vi "Target CSM.vi"(5 "Init State(\"Macro: Initialize\")":string="Macro: Initialize", 7 "Name(\"\" to use uuid)":string="CSM Tiny") -> ()   [LabVIEW 2020]
doc: "Template for building CSM Module without User Interface.\n\n<b>Inputs:</b>\n- <b>Name(\"\" to use uuid)</b>: Module Name\n - If Input is \"\", an uuid will be used for module name. The module is marked as stand-alone mode and will not be included in module list.\n - Fi Input end with '#', the module will worked in worker mode. Modules with the same name will shared the same message queue. Any external message will be processed by one of the modules, depends on who is free.\n - Otherwise, the input string will be used as module name, which should be unique in system. CSM will go to \"Critical Error\" state if duplicated module name is used in system.\n\n<b>Outputs:</b>\n - N/A"
uses:
  <userlib>/_NEVSTOP/Communicable State Machine(CSM)/_Support/Priority Queue/Priority Queue.lvclass/Priority Queue.ctl
  <userlib>/_NEVSTOP/Communicable State Machine(CSM)/AdvanceAPI/CSM - Revert Arguments-Safe String.vi
  <userlib>/_NEVSTOP/Communicable State Machine(CSM)/_Support/Common/Trim Single line Text.vi
  <userlib>/_NEVSTOP/Communicable State Machine(CSM)/AdvanceAPI/CSM - Break Down Multiple States String.vi
  <userlib>/_NEVSTOP/Communicable State Machine(CSM)/AdvanceAPI/CSM - Compact Multiple States.vi
  <userlib>/_NEVSTOP/Communicable State Machine(CSM)/AdvanceAPI/CSM - Make String Arguments Safe.vi
  <userlib>/_NEVSTOP/Communicable State Machine(CSM)/_Support/Process/CSMP-Async Call.vi
  <userlib>/_NEVSTOP/Communicable State Machine(CSM)/_Support/GlobalEvent/GEvt-Generate Status Log.vi
  <userlib>/_NEVSTOP/Communicable State Machine(CSM)/_Support/Process/CSMP-Broadcast.vi
  <userlib>/_NEVSTOP/Communicable State Machine(CSM)/_Support/GlobalEvent/GEvt-Generate Interrupt Log.vi
  <userlib>/_NEVSTOP/Communicable State Machine(CSM)/_Support/GlobalEvent/GEvt-Generate Register Log.vi
  <userlib>/_NEVSTOP/Communicable State Machine(CSM)/_Support/Process/CSMP-Register Status.vi
  <userlib>/_NEVSTOP/Communicable State Machine(CSM)/_Support/GlobalEvent/GEvt-Generate Unregister Log.vi
  <userlib>/_NEVSTOP/Communicable State Machine(CSM)/_Support/Process/CSMP-Unregister Status.vi
  <userlib>/_NEVSTOP/Communicable State Machine(CSM)/_Support/Process/CSMP-Sync Call.vi
  <userlib>/_NEVSTOP/Communicable State Machine(CSM)/_Support/CSMQ/_CSMObj-Unlock.vi
  <userlib>/_NEVSTOP/Communicable State Machine(CSM)/_Support/Process/CSMP-PostPostMsg.vi
  <userlib>/_NEVSTOP/Communicable State Machine(CSM)/_Support/Process/CSMP-PostSendMsg.vi
  <userlib>/_NEVSTOP/Communicable State Machine(CSM)/_Support/CSMQ/_CSMObj-Lock State.vi
  <userlib>/_NEVSTOP/Communicable State Machine(CSM)/_Support/Common/Splite Reason String Part.vi
  <userlib>/_NEVSTOP/Communicable State Machine(CSM)/_Support/CSMQ/_CSMOFGV Release.vi
  <userlib>/_NEVSTOP/Communicable State Machine(CSM)/_Support/Common/Remove Comments from Line.vi
  <userlib>/_NEVSTOP/Communicable State Machine(CSM)/_Support/Common/Splite Single-line Message.vi
  <userlib>/_NEVSTOP/Communicable State Machine(CSM)/_Support/Common/Parse Next Single-line State.vi
  <userlib>/_NEVSTOP/Communicable State Machine(CSM)/_Support/CSMQ/_CSMOFGV Dequeue.vi
  <userlib>/_NEVSTOP/Communicable State Machine(CSM)/_Support/CSMQ/_CSMObj-Log Error if in a Remote Session.vi
  <userlib>/_NEVSTOP/Communicable State Machine(CSM)/_Support/GlobalEvent/GEvt-Generate State Change Log.vi
  <userlib>/_NEVSTOP/Communicable State Machine(CSM)/_Support/GlobalEvent/GEvt-Generate Remaining States Log.vi
  <userlib>/_NEVSTOP/Communicable State Machine(CSM)/_Support/GlobalEvent/GEvt-Generate Module Destroyed Log.vi
  <userlib>/_NEVSTOP/Communicable State Machine(CSM)/_Support/GlobalEvent/GEvt-Generate Complete Log.vi
  <userlib>/_NEVSTOP/Communicable State Machine(CSM)/_Support/GlobalEvent/GEvt-Generate Module Created Log.vi
  <userlib>/_NEVSTOP/Communicable State Machine(CSM)/_Support/GlobalEvent/Cache-GEvt Filter Object.vi
  <userlib>/_NEVSTOP/Communicable State Machine(CSM)/_Support/Common/Format Timestamp.vi
  <userlib>/_NEVSTOP/Communicable State Machine(CSM)/AdvanceAPI/CSM - Keywords.vi
  <userlib>/_NEVSTOP/Communicable State Machine(CSM)/_Support/CSMQ/_CSMObj-Message Check.vi
  <userlib>/_NEVSTOP/Communicable State Machine(CSM)/_Support/CSMQ/_CSMObj-Enqueue Cross-Module Message.vi
  <userlib>/_NEVSTOP/Communicable State Machine(CSM)/_Support/CSMQ/_CSMOFGV Get.vi
  <userlib>/_NEVSTOP/Communicable State Machine(CSM)/_Support/GlobalEvent/GEvt-Generate with Rule Check.vi
  <userlib>/_NEVSTOP/Communicable State Machine(CSM)/_Support/FGV-BroadcastRegistry/Cache-Broadcast Registry Search Result.vi
  <userlib>/_NEVSTOP/Communicable State Machine(CSM)/AdvanceAPI/CSM - Register Status Change.vi
  <userlib>/_NEVSTOP/Communicable State Machine(CSM)/AdvanceAPI/CSM - Unregister Status Change.vi
  <userlib>/_NEVSTOP/Communicable State Machine(CSM)/_Support/Common/Hex Str to U8 Data.vi
  <userlib>/_NEVSTOP/Communicable State Machine(CSM)/_Support/Common/Concatenate State with Arguments.vi
  <userlib>/_NEVSTOP/Communicable State Machine(CSM)/_Support/Common/U8 Data to Hex Str.vi
  <userlib>/_NEVSTOP/Communicable State Machine(CSM)/_Support/Priority Queue/Dequeue Element.vi
  <userlib>/_NEVSTOP/Communicable State Machine(CSM)/_Support/Priority Queue/Enqueue Element.vi
  <userlib>/_NEVSTOP/Communicable State Machine(CSM)/_Support/GlobalEvent/LogFilter/Filter Check.vi
  <userlib>/_NEVSTOP/Communicable State Machine(CSM)/Utility/Trim Both Whitespace.vi
  <userlib>/_NEVSTOP/Communicable State Machine(CSM)/_Support/GlobalEvent/FGV-GlobalEventRef.vi
  <userlib>/_NEVSTOP/Communicable State Machine(CSM)/_Support/GlobalEvent/global-GEvnt Filter Change Flag.vi
  <userlib>/_NEVSTOP/Communicable State Machine(CSM)/FGV-GEvt Filter Obj.vi
  <userlib>/_NEVSTOP/Communicable State Machine(CSM)/_Support/CSMQ/_CSMOFGV Obtain.vi
  <userlib>/_NEVSTOP/Communicable State Machine(CSM)/_Support/GlobalEvent/LogFilter/CheckVIs/Group Check - CSM.vi
  <userlib>/_NEVSTOP/Communicable State Machine(CSM)/_Support/GlobalEvent/LogFilter/CheckVIs/Group Check - LogType.vi
  <userlib>/_NEVSTOP/Communicable State Machine(CSM)/_Support/GlobalEvent/LogFilter/CheckVIs/Group Check - State.vi
  <userlib>/_NEVSTOP/Communicable State Machine(CSM)/_Support/GlobalEvent/LogFilter/CheckVIs/CSM Check - LogType.vi
  <userlib>/_NEVSTOP/Communicable State Machine(CSM)/_Support/GlobalEvent/LogFilter/CheckVIs/CSM Check - State.vi
  <userlib>/_NEVSTOP/Communicable State Machine(CSM)/_Support/GlobalEvent/LogFilter/CheckVIs/CSM Check - StateType.vi
  <userlib>/_NEVSTOP/Communicable State Machine(CSM)/_Support/GlobalEvent/LogFilter/CheckVIs/Group Check - StateType.vi
  <userlib>/_NEVSTOP/Communicable State Machine(CSM)/_Support/CSMQ/_CSMOFGV.vi
  <userlib>/_NEVSTOP/Communicable State Machine(CSM)/_Support/Error/CSM Not Allowed Message.vi
  <userlib>/_NEVSTOP/Communicable State Machine(CSM)/_Support/GlobalEvent/FGV-StatusChangeEventRef.vi
  <userlib>/_NEVSTOP/Communicable State Machine(CSM)/_Support/FGV-BroadcastRegistry/global-CSMQ FGV Change Flag.vi
  <userlib>/_NEVSTOP/Communicable State Machine(CSM)/_Support/FGV-BroadcastRegistry/global-Broadcast Cache Change Flag.vi
  <userlib>/_NEVSTOP/Communicable State Machine(CSM)/_Support/BroadcastRegistry/HelperVI/Broadcast Item Key.vi
  <userlib>/_NEVSTOP/Communicable State Machine(CSM)/_Support/FGV-BroadcastRegistry/FGV-BroadcastRegistry.vi
  <userlib>/_NEVSTOP/Communicable State Machine(CSM)/_Support/Message/Parse Register Message.vi
  <userlib>/_NEVSTOP/Communicable State Machine(CSM)/_Support/Message/Parse Unregister Message.vi
  <userlib>/_NEVSTOP/Communicable State Machine(CSM)/Communicable State Machine.lvlib
panel:
  out "State History":string
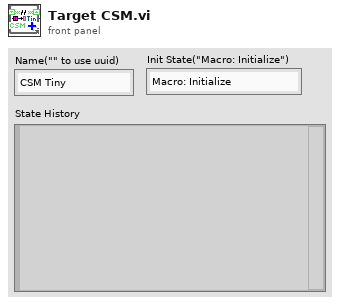
[diagram p1: front panel]
types:
  T1 = enum32{"Invalid", "Standard", "Closed", "Hidden", "Minimized", "Maximized"}
  T2 = enum32{"invalid app kind", "Development System", "Run Time System", "Student Edition", "Embedded LabVIEW", "Evaluation", "Custom"}
  T3 = typedef "Communicable State Machine.lvlib/_CSM_Response Source Message.ctl" = cluster{"‘State":string, "’Arguments":string, "’Error":errorcluster}
  T4 = cluster{"Current VI Reference":refnum<vi>, "Close Panel on Exit?":bool}
  T5 = cluster{"Core":cluster{"Current VI Reference":refnum<vi>, "Close Panel on Exit?":bool}, "Your Boolean data":bool, "Your string data":string}
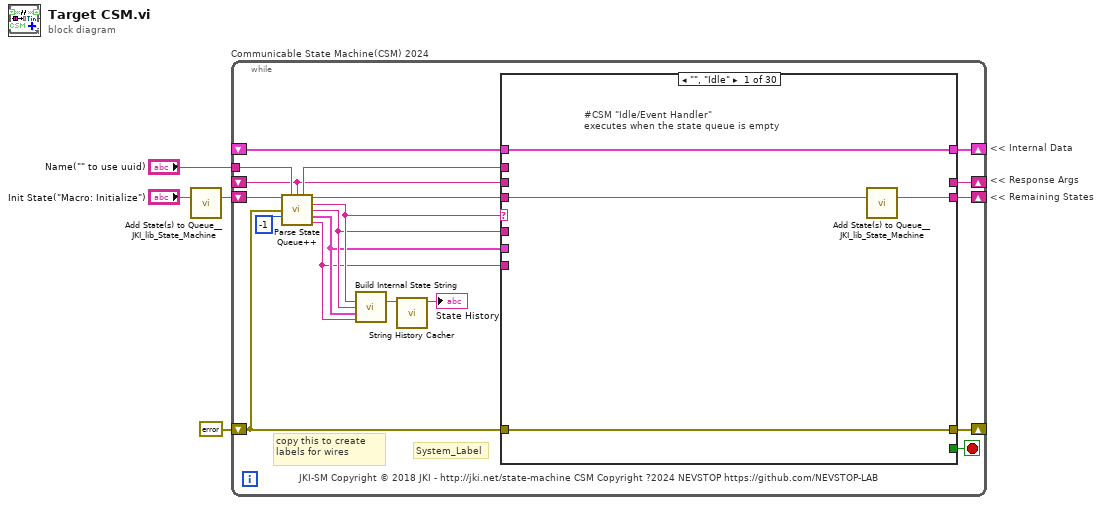
[diagram p0: block diagram]
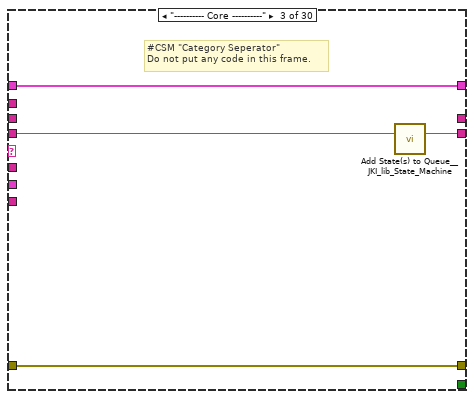
[diagram p3: hidden frame]
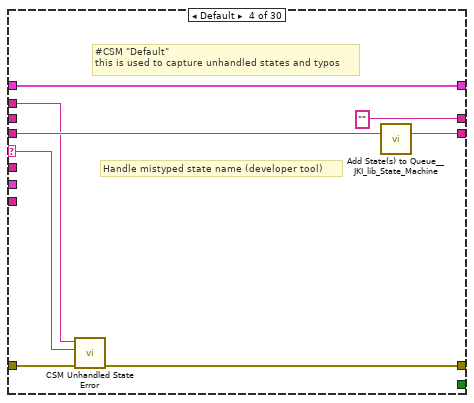
[diagram p4: hidden frame]
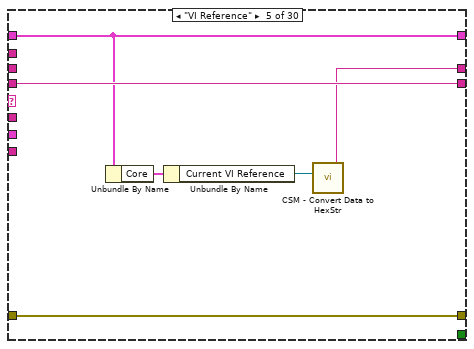
[diagram p5: hidden frame]
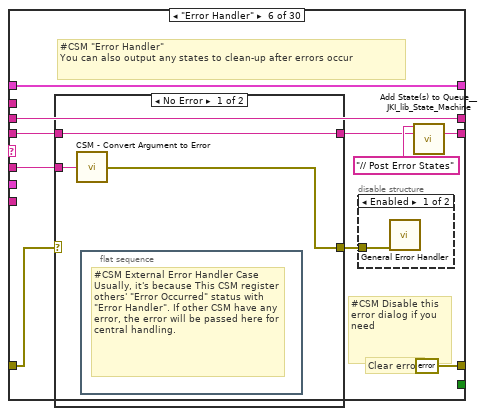
[diagram p6: hidden frame]
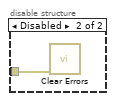
[diagram p7: hidden frame]
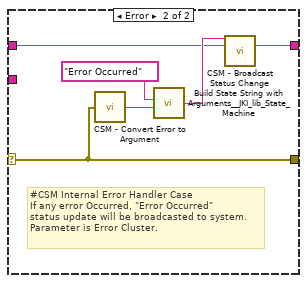
[diagram p8: hidden frame]
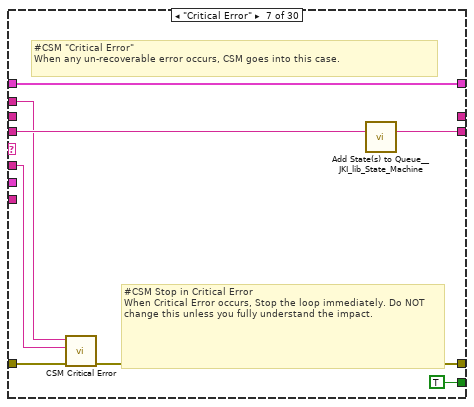
[diagram p9: hidden frame]
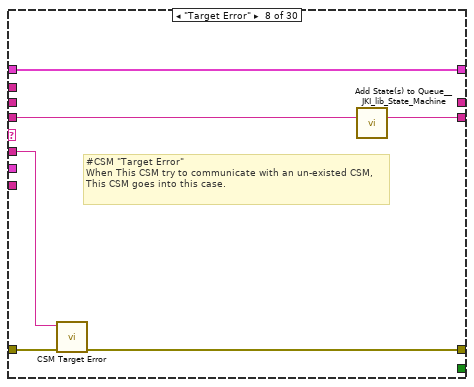
[diagram p10: hidden frame]
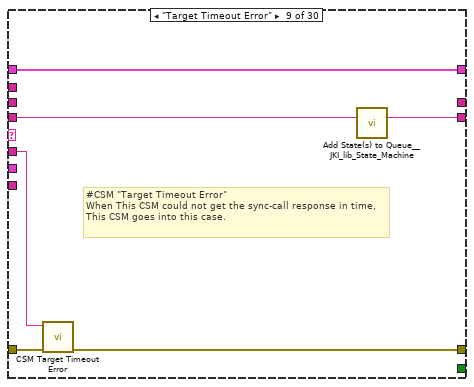
[diagram p11: hidden frame]
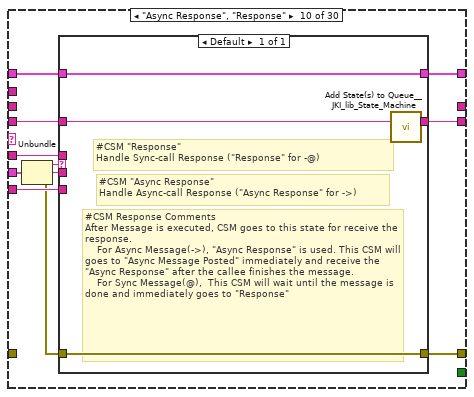
[diagram p12: hidden frame]
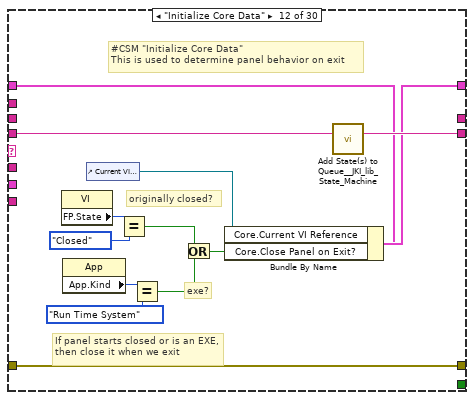
[diagram p14: hidden frame]
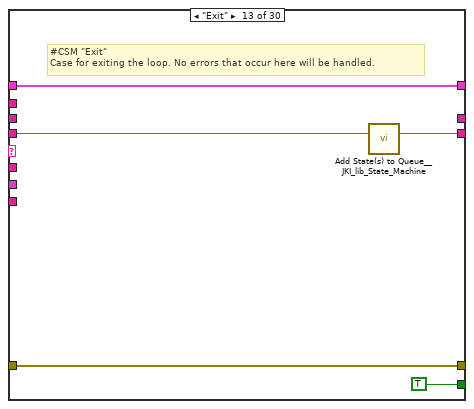
[diagram p15: hidden frame]
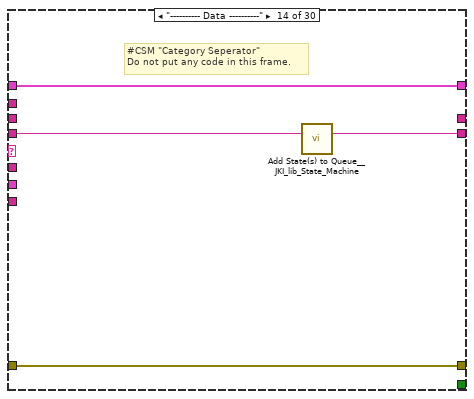
[diagram p16: hidden frame]
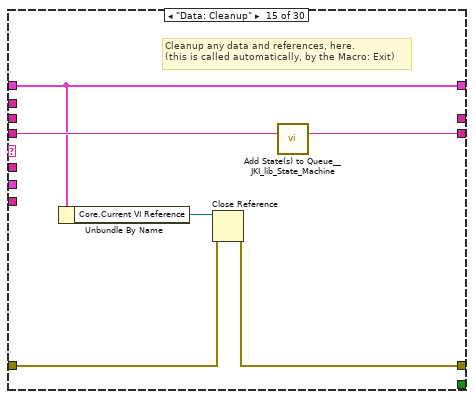
[diagram p17: hidden frame]
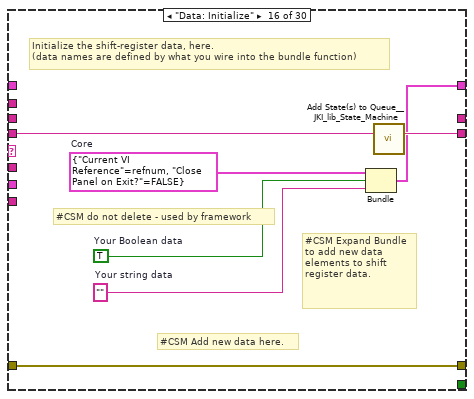
[diagram p18: hidden frame]
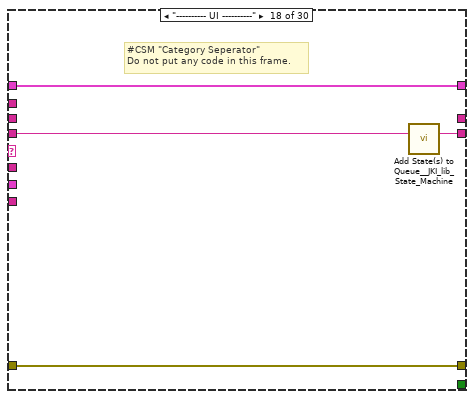
[diagram p20: hidden frame]
diagram:
  # "<< Internal Data"
  # "<< Response Args"
  # "<< Remaining States"
  n1 = call <vilib>:"Add State(s) to Queue__JKI_lib_State_Machine.vi"("State(s) in (\"\")"="Init State(\"Macro: Initialize\")") -> ("States Out"=w4:string)  [unwired: 14 in]
  n2 = while "Communicable State Machine(CSM) 2024" {
    shift-right: [w18] -> _
    shift-left: _ -> [w17]
    shift-right: [w21] -> _
    shift-left: errorcluster {"status"=FALSE, "code"=0, "source"=""} ("error out") -> [w16]
    shift-right: [w20] -> _
    shift-left: w4 -> [w22]
    tunnel: "Name(\"\" to use uuid)" -> [w14]
    shift-right: [w15] -> _
    shift-left: _ -> [w6]
    stop <- w19 stop-if-true
    # "copy this to create labels for wires"
    # "System_Label"
    # "JKI-SM Copyright © 2018 JKI - http://jki.net/state-machine CSM Copyright ?2024 NEVSTOP https://github.com/NEVSTOP-LAB"
    n3 = call <userlib>:"Parse State Queue++.vi"("State Queue"=w22, "Name(\"\" to use uuid)"=w14, "Response Arguments"=w6, "Error In (no error)"=w16, "Dequeue Timeout(0ms)"=-1 ("Timeout")) -> ("Name Used"=w7:string, "Remaining States"=w23:string, "Current State"=w11:string, "Arguments"=w10:string, ">> Response Source Message >>"=w9:T3, ">> Source CSM >>"=w8:string)  [unwired: 5 in]
    n4 = call <userlib>:"Build Internal State String.vi"("State"=w11, "Arguments (\"\")"=w10, ">> Response Source Message >>"=w9, "Source (\"\")"=w8) -> ("State with Arguments"=w12:string)  [unwired: 11 in]
    n5 = call <userlib>:"String History Cacher.vi"("String"=w12) -> ("String Cache"=→"State History":string)  [unwired: 10 in]
    n6 = case shown="\"\", \"Idle\"" w11 {
      selector: w11 -> [_ _ _ w37 _ _ _ _ _ _ _ _ _ _ _ _ _ _ _ _ _ _ _ _ _ _ _ _ _ _]
      tunnel: w23 -> [w24 w29 w34 w41 w47 w54 w75 w81 w87 w95 w106 w120 w125 w129 w135 w142 w144 w149 w153 w159 w174 w243 w248 w255 w257 w262 w268 w273 w277 w281]
      tunnel: w10 -> [_ _ _ _ _ w53 w71 w80 w85 w94 _ _ _ _ _ _ _ _ _ w154 w168 _ _ _ _ w260 _ _ _ _]
      tunnel: w17 -> [w25 w28 w31 w39 w46 w57 w76 w82 w88 w97 w105 w113 w123 w126 w130 _ w143 w146 w151 w157 w170 w240 w245 w252 w256 w261 w267 w270 w274 w278]
      tunnel: [w26 w30 w32 w35 w48 errorcluster {"status"=FALSE, "code"=0, "source"=""} ("error out") w72 w78 w84 w100 w107 w117 w122 w127 w131 w139 w145 w147 w150 w155 w171 w241 w246 w253 w258 w263 w269 w271 w275 w279] -> w21
      tunnel: w16 -> [w26 w30 w32 w42 w48 w55 w77 w79 w86 _ w107 w117 w122 w127 w132 w139 w145 w147 w150 w156 w172 w241 w246 w253 w258 w263 w269 w271 w275 w279]
      tunnel: [w27 w29 w33 w40 w47 w50 w74 w83 w89 w96 w106 w119 w124 w128 w134 w141 w144 w148 w152 w158 w173 w242 w247 w254 w257 w262 w268 w272 w276 w280] -> w20
      tunnel: [_ _ _ _ _ _ TRUE _ _ _ _ _ TRUE _ _ _ _ _ _ _ _ _ _ _ _ _ _ _ _ _] -> w19
      tunnel: [w25 w28 w31 w39 w46 w57 w76 w82 w88 w98 w105 w118 w123 w126 w130 w140 w143 w146 w151 w157 w170 w240 w245 w252 w256 w261 w267 w270 w274 w278] -> w18
      tunnel: w8 -> [_ _ _ _ _ _ _ _ _ w92 _ _ _ _ _ _ _ _ _ _ _ _ _ _ _ _ _ _ _ _]
      tunnel: w9 -> [_ _ _ _ _ _ _ _ _ w99 _ _ _ _ _ _ _ _ _ _ _ _ _ _ _ _ _ _ _ _]
      tunnel: [_ _ _ "" w43 w49 _ _ _ _ _ _ _ _ _ _ _ _ _ _ _ _ _ _ _ w259 "API1 Response" _ _ _] -> w15
      tunnel: w7 -> [_ _ _ w36 _ _ w70 _ _ _ _ _ _ _ _ _ _ _ _ _ _ _ _ _ _ _ _ _ _ _]
      tunnel: w6 -> [_ _ _ _ _ w49 _ _ _ _ _ _ _ _ _ _ _ _ _ _ _ _ _ _ _ _ _ _ _ _]
      frame "", "Idle" {
        # "#CSM \"Idle/Event Handler\"\nexecutes when the state queue is empty"
        n7 = call <vilib>:"Add State(s) to Queue__JKI_lib_State_Machine.vi"("State(s) in (\"\")"=w24) -> ("States Out"=w27:string)  [unwired: 14 in]
      }
      frame "CSM Documentation" {
        # "#CSM README FIRST\n\nCommunicable State Machine(CSM) is a LabVIEW application framework that builds upon JKI State Machine(JKISM). It follows the pattern of JKISM and extends the keywords to describe message communication between modules, including concepts such as Sync-Message, Async-Message, Subscription/Unsubscription of status - essential elements for creating reusable code modules. For more information, please visit the CSM wiki: https://nevstop-lab.github.io/CSM-Wiki/\n\nFor instructions on JKI State Machine, visit: http://jki.net/state-machine/\nFor information about CSM, visit: https://github.com/NEVSTOP-LAB"
        # "#CSM \"Documentation\"\nCase for holding CSM Documenation"
      }
      frame "---------- Core ----------" {
        # "#CSM \"Category Seperator\"\nDo not put any code in this frame."
        n8 = call <vilib>:"Add State(s) to Queue__JKI_lib_State_Machine.vi"("State(s) in (\"\")"=w34) -> ("States Out"=w33:string)  [unwired: 14 in]
      }
      frame Default {
        # "#CSM \"Default\"\nthis is used to capture unhandled states and typos"
        # "Handle mistyped state name (developer tool)"
        n9 = call <userlib>:"CSM Unhandled State Error.vi"("error in (no error)"=w42, "Current State"=w37, "CSM Name"=w36) -> ("error out"=w35:errorcluster)  [unwired: 8 in]
        n10 = call <vilib>:"Add State(s) to Queue__JKI_lib_State_Machine.vi"("State(s) in (\"\")"=w41) -> ("States Out"=w40:string)  [unwired: 14 in]
      }
      frame "VI Reference" {
        n11 = Unbundle By Name(w46) -> ("Core"=w45:T4)
        n12 = Unbundle By Name(w45) -> ("Current VI Reference"=w44:refnum<vi>)
        n13 = call <userlib>:"CSM - Convert Data to HexStr.vi"("Variant"=w44) -> ("HEX String (0-9,A-F)"=w43:string)  [unwired: 8 in]
      }
      frame "Error Handler" {
        # "#CSM Disable this error dialog if you need"
        # "#CSM \"Error Handler\"\nYou can also output any states to clean-up after errors occur"
        # "Clear error"
        n14 = case shown="No Error" w55 {
          selector: w55 -> [_ w64]
          tunnel: [w63 w66] -> w51
          tunnel: w54 -> [w63 w65]
          tunnel: w53 -> [w62 _]
          tunnel: [w61 w64] -> w56
          frame No Error {
            n15 = call <userlib>:"CSM - Convert Argument to Error.vi"("Argument"=w62) -> ("error"=w61:errorcluster)  [unwired: 4 in]
            n16 = flat-sequence {
              frame #0 {
                # "#CSM External Error Handler Case\nUsually, it's because This CSM register others' \"Error Occurred\" status with \"Error Handler\". If other CSM have any error, the error will be passed here for central handling."
              }
            }
          }
          frame Error {
            # "#CSM Internal Error Handler Case \nIf any error Occurred, \"Error Occurred\" \nstatus update will be broadcasted to system.\nParameter is Error Cluster."
            n17 = call <userlib>:"CSM - Convert Error to Argument.vi"("error in (no error)"=w64) -> ("Arguments"=w68:string)  [unwired: 4 in]
            n18 = call <vilib>:"Build State String with Arguments__JKI_lib_State_Machine.vi"("Arguments (\"\")"=w68, "State"="Error Occurred" ("Status with Arguments")) -> ("State with Arguments"=w67:string)  [unwired: 4 in]
            n19 = call <userlib>:"CSM - Broadcast Status Change.vi"("Status with Arguments"=w67, "State Queue"=w65) -> ("Remaining States"=w66:string)  [unwired: 13 in]
          }
        }
        n20 = disable-structure shown="Enabled" {
          disable-tunnel: w56 -> [w59 w60]
          frame Enabled {
            n21 = call <vilib>:"General Error Handler.vi"("error in (no error)"=w59) -> ()  [unwired: 10 in, 5 out]
          }
          frame Disabled {
            n22 = call <vilib>:"Clear Errors.vi"("error in (no error)"=w60) -> ()  [unwired: 5 in, 2 out]
          }
        }
        n23 = call <vilib>:"Add State(s) to Queue__JKI_lib_State_Machine.vi"("State(s) in Front (\"\")"="// Post Error States", "State(s) in (\"\")"=w51) -> ("States Out"=w50:string)  [unwired: 13 in]
      }
      frame "Critical Error" {
        # "#CSM Stop in Critical Error\nWhen Critical Error occurs, Stop the loop immediately. Do NOT change this unless you fully understand the impact."
        # "#CSM \"Critical Error\"\nWhen any un-recoverable error occurs, CSM goes into this case."
        n24 = call <userlib>:"CSM Critical Error.vi"("error in (no error)"=w77, "Arugments(as Reason)"=w71, "CSM Name"=w70) -> ("error out"=w72:errorcluster)  [unwired: 8 in]
        n25 = call <vilib>:"Add State(s) to Queue__JKI_lib_State_Machine.vi"("State(s) in (\"\")"=w75) -> ("States Out"=w74:string)  [unwired: 14 in]
      }
      frame "Target Error" {
        # "#CSM \"Target Error\"\nWhen This CSM try to communicate with an un-existed CSM, This CSM goes into this case."
        n26 = call <userlib>:"CSM Target Error.vi"("error in (no error)"=w79, "Arguments(as CSM Name)"=w80) -> ("error out"=w78:errorcluster)  [unwired: 9 in]
        n27 = call <vilib>:"Add State(s) to Queue__JKI_lib_State_Machine.vi"("State(s) in (\"\")"=w81) -> ("States Out"=w83:string)  [unwired: 14 in]
      }
      frame "Target Timeout Error" {
        # "#CSM \"Target Timeout Error\"\nWhen This CSM could not get the sync-call response in time, This CSM goes into this case."
        n28 = call <userlib>:"CSM Target Timeout Error.vi"("error in (no error)"=w86, "Arguments(as CSM Name)"=w85) -> ("error out"=w84:errorcluster)  [unwired: 9 in]
        n29 = call <vilib>:"Add State(s) to Queue__JKI_lib_State_Machine.vi"("State(s) in (\"\")"=w87) -> ("States Out"=w89:string)  [unwired: 14 in]
      }
      frame "Async Response", "Response" {
        n30 = Unbundle(w99) -> ("‘State"=w93:string, "’Arguments"=w91:string, "’Error"=w90:errorcluster)
        n31 = case shown="Default" w93 {
          tunnel: [w104] -> w100
          tunnel: w90 -> [w104]
          tunnel: [w103] -> w98
          tunnel: w97 -> [w103]
          tunnel: [w101] -> w96
          tunnel: w95 -> [w102]
          tunnel: w94 -> [_]
          tunnel: w92 -> [_]
          tunnel: w91 -> [_]
          frame Default {
            # "#CSM Response Comments\nAfter Message is executed, CSM goes to this state for receive the response.\n    For Async Message(->), \"Async Response\" is used. This CSM will goes to \"Async Message Posted\" immediately and receive the \"Async Response\" after the callee finishes the message.\n    For Sync Message(@),  This CSM will wait until the message is done and immediately goes to \"Response\""
            # "#CSM \"Async Response\"\nHandle Async-call Response (\"Async Response\" for ->)"
            # "#CSM \"Response\"\nHandle Sync-call Response (\"Response\" for -@)"
            n32 = call <vilib>:"Add State(s) to Queue__JKI_lib_State_Machine.vi"("State(s) in (\"\")"=w102) -> ("States Out"=w101:string)  [unwired: 14 in]
          }
        }
      }
      frame "Async Message Posted" {
        # "a"
        # "a"
        # "a"
        # "a"
        # "a"
        # "a"
        # "a"
        # "a"
        # "a"
        # "a"
        # "a"
        # "a"
        # "a"
        # "a"
        # "a"
        # "a"
        # "a"
        # "a"
        # "a"
        # "a"
        # "a"
        # "a"
        # "a"
        # "a"
        # "a"
        # "a"
        # "a"
        # "a"
        # "a"
        # "a"
        # "a"
        # "a"
        # "a"
        # "a"
        # "a"
        # "a"
        # "a"
        # "a"
        # "a"
        # "a"
        # "a"
        # "a"
        # "a"
        # "a"
        # "a"
        # "a"
        # "a"
        # "a"
        # "a"
        # "a"
        # "a"
        # "a"
        # "a"
        # "a"
        # "a"
        # "a"
        # "a"
        # "a"
        # "a"
        # "a"
        # "a"
        # "a"
        # "a"
        # "a"
        # "a"
        # "a"
        # "a"
        # "a"
        # "a"
        # "a"
        # "a"
        # "a"
        # "a"
        # "a"
        # "a"
        # "a"
        # "a"
        # "a"
        # "a"
        # "a"
        # "a"
        # "a"
        # "a"
        # "a"
        # "a"
        # "a"
        # "a"
        # "a"
        # "a"
        # "a"
        # "a"
        # "a"
        # "a"
        # "a"
        # "a"
        # "a"
        # "a"
        # "a"
        # "a"
        # "a"
        # "a"
        # "a"
        # "a"
        # "a"
        # "a"
        # "a"
        # "a"
        # "a"
        # "a"
        # "a"
        # "a"
        # "a"
        # "a"
        # "a"
        # "a"
        # "a"
        # "a"
        # "a"
        # "a"
        # "a"
        # "a"
        # "a"
        # "a"
        # "a"
        # "a"
        # "a"
        # "a"
        # "a"
        # "a"
        # "a"
        # "a"
        # "a"
        # "a"
        # "a"
        # "a"
        # "a"
        # "a"
        # "a"
        # "a"
        # "a"
        # "a"
        # "a"
        # "a"
        # "a"
        # "a"
        # "a"
        # "a"
        # "a"
        # "a"
        # "a"
        # "a"
        # "a"
        # "a"
        # "a"
        # "a"
        # "a"
        # "a"
        # "a"
        # "a"
        # "a"
        # "a"
        # "a"
        # "a"
        # "a"
        # "a"
        # "a"
        # "a"
        # "a"
        # "a"
        # "a"
        # "a"
        # "a"
        # "a"
        # "a"
        # "a"
        # "a"
        # "a"
        # "a"
        # "a"
        # "a"
        # "a"
        # "a"
        # "a"
        # "a"
        # "a"
        # "a"
        # "a"
        # "a"
        # "a"
        # "a"
        # "a"
        # "a"
        # "a"
        # "a"
        # "a"
        # "a"
        # "a"
        # "a"
        # "a"
        # "a"
        # "a"
        # "a"
        # "a"
        # "a"
        # "a"
        # "a"
        # "a"
        # "a"
        # "a"
        # "a"
        # "a"
        # "a"
        # "a"
        # "a"
        # "a"
        # "a"
        # "a"
        # "a"
        # "a"
        # "a"
        # "a"
        # "a"
        # "a"
        # "a"
        # "a"
        # "a"
        # "a"
        # "a"
        # "a"
        # "a"
        # "a"
        # "a"
        # "a"
        # "a"
        # "a"
        # "a"
        # "a"
        # "a"
        # "a"
        # "a"
        # "a"
        # "a"
        # "a"
        # "a"
        # "a"
        # "a"
        # "a"
        # "a"
        # "a"
        # "a"
        # "a"
        # "a"
        # "a"
        # "a"
        # "a"
        # "a"
        # "a"
        # "a"
        # "a"
        # "a"
        # "a"
        # "a"
        # "a"
        # "a"
        # "a"
        # "a"
        # "a"
        # "a"
        # "a"
        # "a"
        # "a"
        # "a"
        # "a"
        # "a"
        # "a"
        # "a"
        # "a"
        # "a"
        # "a"
        # "a"
        # "a"
        # "a"
        # "a"
        # "a"
        # "a"
        # "a"
        # "a"
        # "a"
        # "a"
        # "a"
        # "a"
        # "a"
        # "a"
        # "a"
        # "a"
        # "a"
        # "a"
        # "a"
        # "a"
        # "a"
        # "a"
        # "a"
        # "a"
        # "a"
        # "a"
        # "a"
        # "a"
        # "a"
        # "a"
        # "a"
        # "a"
        # "a"
        # "a"
        # "a"
        # "a"
        # "a"
        # "a"
        # "a"
        # "a"
        # "a"
        # "a"
        # "a"
        # "a"
        # "a"
        # "a"
        # "a"
        # "a"
        # "a"
        # "a"
        # "a"
        # "a"
        # "a"
        # "a"
        # "a"
        # "a"
        # "a"
        # "a"
        # "a"
        # "a"
        # "a"
        # "a"
        # "a"
        # "a"
        # "a"
        # "a"
        # "a"
        # "a"
        # "a"
        # "a"
        # "a"
        # "a"
        # "a"
        # "a"
        # "a"
        # "a"
        # "a"
        # "a"
        # "a"
        # "a"
        # "a"
        # "a"
        # "a"
        # "a"
        # "a"
        # "a"
        # "a"
        # "a"
        # "a"
        # "a"
        # "a"
        # "a"
        # "a"
        # "a"
        # "a"
        # "a"
        # "a"
        # "a"
        # "a"
      }
      frame "Initialize Core Data" {
        # "#CSM \"Initialize Core Data\"\nThis is used to determine panel behavior on exit"
        # "originally closed?"
        # "exe?"
        # "If panel starts closed or is an EXE, then close it when we exit"
        n33 = property class="VI"() -> ("FP.State"=w110:T1)  [unwired: 2 in, 2 out]
        n34 = property class="App"() -> ("App.Kind"=w116:T2)  [unwired: 2 in, 2 out]
        n35 = control-ref of="Current VI Reference"() -> (w111:refnum<vi>)
        n36 = Equal?(x=w110, y=T1."Closed" ("Front Panel Window:State")) -> (x = y?=w108:bool)
        n37 = Equal?(x=w116, y=T2."Run Time System" ("Application:Kind")) -> (x = y?=w114:bool)
        n38 = Or(x=w108, y=w114) -> (x .or. y?=w112:bool)
        n39 = Bundle By Name(cluster=w113, "Core.Current VI Reference"=w111, "Core.Close Panel on Exit?"=w112) -> (w118:T5)
        n40 = call <vilib>:"Add State(s) to Queue__JKI_lib_State_Machine.vi"("State(s) in (\"\")"=w120) -> ("States Out"=w119:string)  [unwired: 14 in]
      }
      frame "Exit" {
        # "#CSM \"Exit\"\nCase for exiting the loop. No errors that occur here will be handled."
        n41 = call <vilib>:"Add State(s) to Queue__JKI_lib_State_Machine.vi"("State(s) in (\"\")"=w125) -> ("States Out"=w124:string)  [unwired: 14 in]
      }
      frame "---------- Data ----------" {
        # "#CSM \"Category Seperator\"\nDo not put any code in this frame."
        n42 = call <vilib>:"Add State(s) to Queue__JKI_lib_State_Machine.vi"("State(s) in (\"\")"=w129) -> ("States Out"=w128:string)  [unwired: 14 in]
      }
      frame "Data: Cleanup" {
        # "Cleanup any data and references, here.\n(this is called automatically, by the Macro: Exit)"
        n43 = Unbundle By Name(w130) -> ("Core.Current VI Reference"=w133:refnum<vi>)
        n44 = Close Reference(reference=w133, error in (no error)=w132) -> (error out=w131:errorcluster)
        n45 = call <vilib>:"Add State(s) to Queue__JKI_lib_State_Machine.vi"("State(s) in (\"\")"=w135) -> ("States Out"=w134:string)  [unwired: 14 in]
      }
      frame "Data: Initialize" {
        w136 = T4 {"Current VI Reference"=refnum, "Close Panel on Exit?"=FALSE}  # Core
        w138 = TRUE  # Your Boolean data
        w137 = ""  # Your string data
        # "#CSM do not delete - used by framework"
        # "#CSM Expand Bundle to add new data elements to shift register data."
        # "#CSM Add new data here."
        # "Initialize the shift-register data, here.\n(data names are defined by what you wire into the bundle function)"
        n46 = Bundle("Core"=w136, "Your Boolean data"=w138, "Your string data"=w137) -> (w140:T5)  [unwired: 1 in]
        n47 = call <vilib>:"Add State(s) to Queue__JKI_lib_State_Machine.vi"("State(s) in (\"\")"=w142) -> ("States Out"=w141:string)  [unwired: 14 in]
      }
      frame "Data: Update Indicators" {
      }
      frame "---------- UI ----------" {
        # "#CSM \"Category Seperator\"\nDo not put any code in this frame."
        n48 = call <vilib>:"Add State(s) to Queue__JKI_lib_State_Machine.vi"("State(s) in (\"\")"=w149) -> ("States Out"=w148:string)  [unwired: 14 in]
      }
      frame "UI: Initialize" {
        # "#CSM \"UI: Initialize\"\nInitialize the User Interface, here.\n(this is called automatically, by the Macro: Init)"
        n49 = call <vilib>:"Add State(s) to Queue__JKI_lib_State_Machine.vi"("State(s) in (\"\")"=w153) -> ("States Out"=w152:string)  [unwired: 14 in]
      }
      frame "UI: Cursor Set" {
        # "#CSM \"UI: Cursor Set\"\nSet and Unset Cursor Busy.\n(Usage: \"UI: Cursor Set >> Busy|Idle\")"
        # "Argument"
        n50 = disable-structure shown="Default" {
          disable-tunnel: w156 -> [w162 w167]
          disable-tunnel: [w161 w167] -> w155
          disable-tunnel: w154 -> [w160 _]
          frame condition #0 (active) {
            n51 = case shown="\"Idle\", Default" w160 {
              tunnel: w162 -> [w164 w166]
              tunnel: [w163 w165] -> w161
              frame "Idle", Default {
                n52 = call <vilib>:"Unset Busy.vi"("error in (no error)"=w164) -> ("error out"=w163:errorcluster)  [unwired: 10 in]
              }
              frame "Busy" {
                n53 = call <vilib>:"Set Busy.vi"("error in (no error)"=w166) -> ("error out"=w165:errorcluster)  [unwired: 9 in, 1 out]
              }
            }
          }
          frame condition #1 {
          }
        }
        n54 = call <vilib>:"Add State(s) to Queue__JKI_lib_State_Machine.vi"("State(s) in (\"\")"=w159) -> ("States Out"=w158:string)  [unwired: 14 in]
      }
      frame "UI: Front Panel State" {
        # "#CSM \"UI: Front Panel State\"\nSet Front Panel Open or Closed\n(Usage: \"UI: Front Panel State >> Open|Close\")"
        # "Argument"
        n55 = Unbundle By Name(w170) -> ("Core.Current VI Reference"=w169:refnum<vi>)
        n56 = call <vilib>:"Add State(s) to Queue__JKI_lib_State_Machine.vi"("State(s) in (\"\")"=w174) -> ("States Out"=w173:string)  [unwired: 14 in]
        n57 = case shown="\"Close\", \"Closed\"" w168 {
          tunnel: w172 -> [w180 w195 w206 w219 w232]
          tunnel: [w182 w196 w208 w221 w234] -> w171
          tunnel: w169 -> [w181 w193 w207 w220 w233]
          frame "Open", "Standard", Default {
            w175 = T1."Standard" ("State")
            n58 = property class="VI"(reference=w181, error in=w180) -> (reference out=w178:refnum<vi>, error out=w179:errorcluster, "FP.State"=w177:T1)
            n59 = Not Equal?(x=w177, y=w175) -> (x != y?=w176:bool)
            n60 = case shown="True" w176 {
              tunnel: [w186 w188] -> w182
              tunnel: w179 -> [w185 w188]
              tunnel: w178 -> [w184 _]
              tunnel: w175 -> [w183 _]
              frame True {
                n61 = invoke class="VI" method="FP.Open"(reference=w184, error in=w185, "Activate"=TRUE, "State"=w183) -> (error out=w186:errorcluster)  [unwired: 1 in, 4 out]
              }
              frame False {
              }
            }
          }
          frame "Close", "Closed" {
            n62 = property class="VI"(reference=w193, error in=w195) -> (reference out=w192:refnum<vi>, error out=w194:errorcluster, "FP.State"=w190:T1)
            n63 = Not Equal?(x=w190, y=T1."Closed" ("Front Panel Window:State")) -> (x != y?=w189:bool)
            n64 = case shown="False" w189 {
              tunnel: [w197 w200] -> w196
              tunnel: w194 -> [w197 w199]
              tunnel: w192 -> [_ w198]
              frame False {
              }
              frame True {
                n65 = invoke class="VI" method="FP.Close"(reference=w198, error in=w199) -> (error out=w200:errorcluster)  [unwired: 1 in, 2 out]
              }
            }
          }
          frame "Hidden", "Hide" {
            w201 = T1."Hidden" ("State")
            n66 = property class="VI"(reference=w207, error in=w206) -> (reference out=w204:refnum<vi>, error out=w205:errorcluster, "FP.State"=w203:T1)
            n67 = Not Equal?(x=w203, y=w201) -> (x != y?=w202:bool)
            n68 = case shown="True" w202 {
              tunnel: [w212 w213] -> w208
              tunnel: w205 -> [w211 w213]
              tunnel: w204 -> [w210 _]
              tunnel: w201 -> [w209 _]
              frame True {
                n69 = invoke class="VI" method="FP.Open"(reference=w210, error in=w211, "State"=w209) -> (error out=w212:errorcluster)  [unwired: 2 in, 4 out]
              }
              frame False {
              }
            }
          }
          frame "Minimize", "Minimized" {
            w214 = T1."Minimized" ("State")
            n70 = property class="VI"(reference=w220, error in=w219) -> (reference out=w217:refnum<vi>, error out=w218:errorcluster, "FP.State"=w216:T1)
            n71 = Not Equal?(x=w216, y=w214) -> (x != y?=w215:bool)
            n72 = case shown="True" w215 {
              tunnel: [w225 w226] -> w221
              tunnel: w218 -> [w224 w226]
              tunnel: w217 -> [w223 _]
              tunnel: w214 -> [w222 _]
              frame True {
                n73 = invoke class="VI" method="FP.Open"(reference=w223, error in=w224, "State"=w222) -> (error out=w225:errorcluster)  [unwired: 2 in, 4 out]
              }
              frame False {
              }
            }
          }
          frame "Maximize", "Maximized" {
            w227 = T1."Maximized" ("State")
            n74 = property class="VI"(reference=w233, error in=w232) -> (reference out=w230:refnum<vi>, error out=w231:errorcluster, "FP.State"=w229:T1)
            n75 = Not Equal?(x=w229, y=w227) -> (x != y?=w228:bool)
            n76 = case shown="True" w228 {
              tunnel: [w238 w239] -> w234
              tunnel: w231 -> [w237 w239]
              tunnel: w230 -> [w236 _]
              tunnel: w227 -> [w235 _]
              frame True {
                n77 = invoke class="VI" method="FP.Open"(reference=w236, error in=w237, "State"=w235) -> (error out=w238:errorcluster)  [unwired: 2 in, 4 out]
              }
              frame False {
              }
            }
          }
        }
      }
      frame "---------- Macro ----------" {
        # "#CSM \"Category Seperator\"\nDo not put any code in this frame."
        n78 = call <vilib>:"Add State(s) to Queue__JKI_lib_State_Machine.vi"("State(s) in (\"\")"=w243) -> ("States Out"=w242:string)  [unwired: 14 in]
      }
      frame "Macro: Initialize" {
        # "#CSM \"Macro: Initialize\"\nInitialization Macro (This is called once, when the VI starts)"
        n79 = call <vilib>:"Add State(s) to Queue__JKI_lib_State_Machine.vi"("State(s) in Front (\"\")"="Data: Initialize\nInitialize Core Data\nData: Update Indicators", "State(s) in (\"\")"=w248) -> ("States Out"=w247:string)  [unwired: 13 in]
      }
      frame "Macro: Exit" {
        # "#CSM \"Macro: Exit\"\nExit Macro (This is called once, when the VI exits)"
        n80 = call <vilib>:"Add State(s) to Queue__JKI_lib_State_Machine.vi"("State(s) in Front (\"\")"="//Exit Sub-Modules ", "State(s) at Back (\"\")"="Data: Cleanup\nExit") -> ("States Out"=w250:string)  [unwired: 13 in]
        n81 = call <vilib>:"Add State(s) to Queue__JKI_lib_State_Machine.vi"("State(s) in Front (\"\")"=w250, "State(s) in (\"\")"=w255) -> ("States Out"=w254:string)  [unwired: 13 in]
      }
      frame "---------- API ----------" {
        # "#CSM \"Category Seperator\"\nDo not put any code in this frame."
      }
      frame "API: API2" {
        # "#CSM API Example\nCopy/Rename this case for your own API"
        # "unpack Hex String  to Variant\nif complex parameter is needed."
        n82 = call <userlib>:"CSM - Convert HexStr to Data.vi"("HEX String"=w260) -> ()  [unwired: 7 in, 2 out]
        n83 = disable-structure shown="Disabled" {
          disable-tunnel: [w264 "API2 Response"] -> w259
          frame Disabled {
            # "pack variant to hexstr \nif complex response is needed."
            # "complex Response"
            n84 = call <userlib>:"CSM - Convert Data to HexStr.vi"() -> ("HEX String (0-9,A-F)"=w264:string)  [unwired: 9 in]
          }
          frame Enabled {
          }
        }
      }
      frame "API: API1" {
        # "#CSM API Example\nCopy/Rename this case for your own API"
        # "#CSM Response\nConnect this to return the response of your API"
        # "#CSM >> Source CSM >>\nIf you need to tell who triggered this state , use this string. If it's this case itself, this string is \"\"."
        # "#CSM >> Arguments >>\nDeal with the parameter if any"
      }
      frame "---------- Action ----------" {
        # "#CSM \"Category Seperator\"\nDo not put any code in this frame."
        n85 = call <vilib>:"Add State(s) to Queue__JKI_lib_State_Machine.vi"("State(s) in (\"\")"=w273) -> ("States Out"=w272:string)  [unwired: 14 in]
      }
      frame "Action: action1" {
        # "#CSM \"Internal State\"\nThis category is used for holding internal states"
        n86 = call <vilib>:"Add State(s) to Queue__JKI_lib_State_Machine.vi"("State(s) in (\"\")"=w277) -> ("States Out"=w276:string)  [unwired: 14 in]
      }
      frame "Action: action2" {
        # "#CSM \"Internal State\"\nThis category is used for holding internal states"
        n87 = call <vilib>:"Add State(s) to Queue__JKI_lib_State_Machine.vi"("State(s) in (\"\")"=w281) -> ("States Out"=w280:string)  [unwired: 14 in]
      }
    }
  }
